vi "auto avance ralentir.vi"(9 "vitesse gauche":dbl, 10 "temps":dbl, 11 "temps de changement de direction":dbl) -> ()   [LabVIEW 2015]
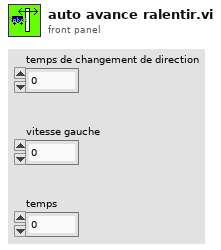
[diagram p1: front panel]
types:
  T1 = typedef "WPI_ServoDeviceRef.ctl" = cluster{"DeviceStatus":errorcluster, "PWM Channel":T2, "DeadBand":T3}
  T2 = typedef "FPGA_DIOPWMChannel.ctl" = enum8{"PWM 0", "PWM 1", "PWM 2", "PWM 3", "PWM 4", "PWM 5", "PWM 6", "PWM 7", "PWM 8", "PWM 9", "PWM MXP 0", "PWM MXP 1", "PWM MXP 2", "PWM MXP 3", "PWM MXP 4", "PWM MXP 5", "PWM MXP 6", "PWM MXP 7", "PWM MXP 8", "PWM MXP 9", "Invalid"}
  T3 = typedef "WPI_PWMDeadband.ctl" = cluster{"Name":string, "maxPositivePwm":i32, "minPositivePwm":i32, "centerPwm":i32, "maxNegativePwm":i32, "minNegativePwm":i32, "angularRange":u16}
  T4 = typedef "WPI_EncoderDevRef.ctl" = cluster{"DevStatus":errorcluster, "EncoderIndex":T5, "CounterIndex":T6, "DistancePerCount":dbl, "Decoding Type":T7}
  T5 = typedef "FPGA_EncoderIdx.ctl" = enum8{"Enc 0", "Enc 1", "Enc 2", "Enc 3", "Enc 4", "Enc 5", "Enc 6", "Enc 7", "Invalid"}
  T6 = typedef "FPGA_CounterCtrSystemIndex.ctl" = enum8{"Ctr 0", "Ctr 1", "Ctr 2", "Ctr 3", "Ctr 4", "Ctr 5", "Ctr 6", "Ctr 7", "Invalid"}
  T7 = typedef "WPI_EncoderType.ctl" = enum16{"1x", "2x", "4x"}
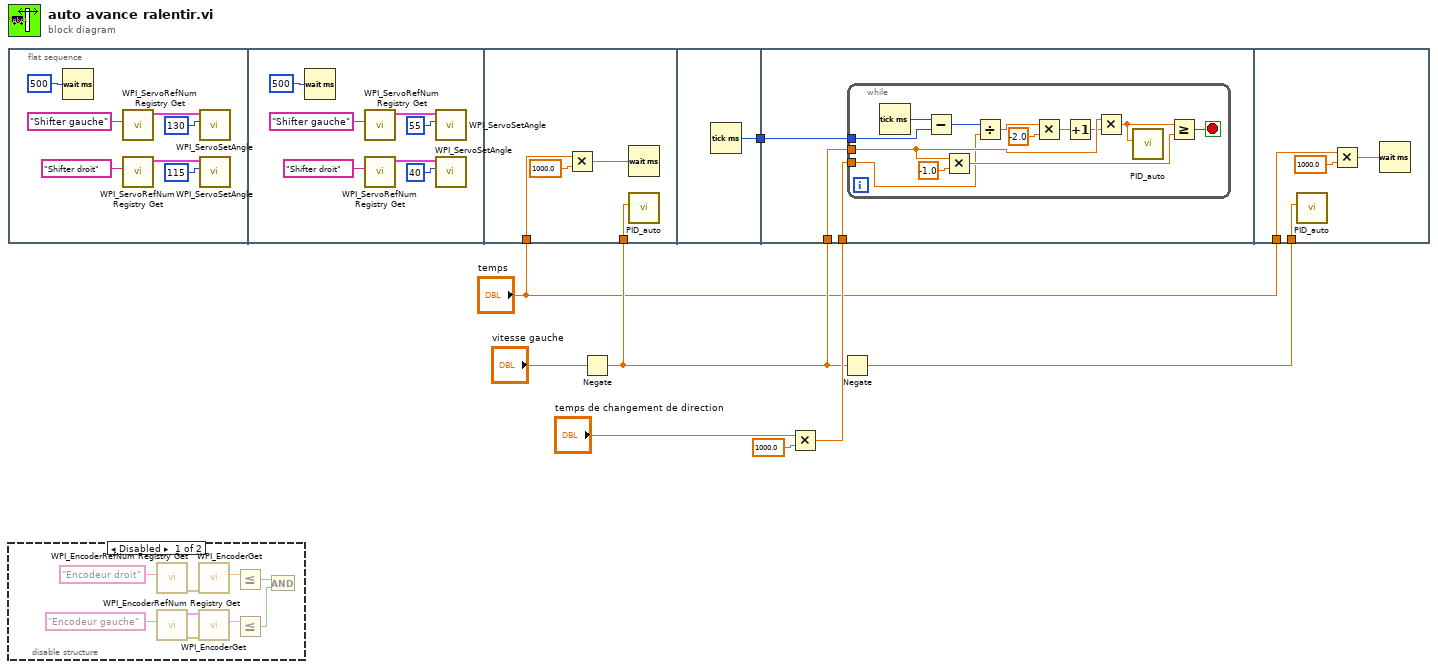
[diagram p0: block diagram]
diagram:
  n1 = flat-sequence {
    tunnel: w3 -> [w26]
    tunnel: "temps" -> [w24]
    tunnel: [w27] -> w8
    tunnel: w8 -> [w30]
    tunnel: w3 -> [w29]
    tunnel: w5 -> [w28]
    tunnel: w2 -> [w47]
    tunnel: "temps" -> [w44]
    frame #0 {
      n2 = Wait (ms)(milliseconds to wait=u32 500) -> ()  [unwired: 1 out]
      n3 = call <vilib>:"WPI_ServoRefNum Registry Get.vi"("refnum name"="Shifter gauche") -> ("ServoDeviceRef"=w14:T1)  [unwired: 9 in, 1 out]
      n4 = call <vilib>:"WPI_ServoRefNum Registry Get.vi"("refnum name"="Shifter droit") -> ("ServoDeviceRef"=w15:T1)  [unwired: 9 in, 1 out]
      n5 = call <vilib>:"WPI_ServoSetAngle.vi"("Angle"=130, "ServoDeviceRef"=w14) -> ()  [unwired: 8 in, 2 out]
      n6 = call <vilib>:"WPI_ServoSetAngle.vi"("Angle"=115, "ServoDeviceRef"=w15) -> ()  [unwired: 8 in, 2 out]
    }
    frame #1 {
      n7 = Wait (ms)(milliseconds to wait=u32 500) -> ()  [unwired: 1 out]
      n8 = call <vilib>:"WPI_ServoRefNum Registry Get.vi"("refnum name"="Shifter gauche") -> ("ServoDeviceRef"=w21:T1)  [unwired: 9 in, 1 out]
      n9 = call <vilib>:"WPI_ServoRefNum Registry Get.vi"("refnum name"="Shifter droit") -> ("ServoDeviceRef"=w22:T1)  [unwired: 9 in, 1 out]
      n10 = call <vilib>:"WPI_ServoSetAngle.vi"("Angle"=55, "ServoDeviceRef"=w21) -> ()  [unwired: 8 in, 2 out]
      n11 = call <vilib>:"WPI_ServoSetAngle.vi"("Angle"=40, "ServoDeviceRef"=w22) -> ()  [unwired: 8 in, 2 out]
    }
    frame #2 {
      n12 = Multiply(x=w24, y=1000.0) -> (x*y=w23:dbl)
      n13 = Wait (ms)(milliseconds to wait=w23) -> ()  [unwired: 1 out]
      n14 = call "PID_auto.vi"("vitesse voulu"=w26) -> ()  [unwired: 11 in]
    }
    frame #3 {
      n15 = Tick Count (ms)() -> (millisecond timer value=w27:u32)
    }
    frame #4 {
      n16 = while {
        tunnel: w30 -> [w34]
        tunnel: w29 -> [w42]
        tunnel: w28 -> [w40]
        stop <- w31 stop-if-true
        n17 = Tick Count (ms)() -> (millisecond timer value=w33:u32)
        n18 = Subtract(x=w33, y=w34) -> (x-y=w39:u32)
        n19 = Multiply(x=w42, y=-1.0) -> (x*y=w41:dbl)
        n20 = Divide(x=w39, y=w40) -> (x/y=w37:dbl)
        n21 = Multiply(x=w37, y=-2.0) -> (x*y=w36:dbl)
        n22 = Increment(x=w36) -> (x+1=w35:dbl)
        n23 = Multiply(x=w42, y=w35) -> (x*y=w32:dbl)
        n24 = call "PID_auto.vi"("vitesse voulu"=w32) -> ()  [unwired: 11 in]
        n25 = Greater Or Equal?(x=w32, y=w41) -> (x >= y?=w31:bool)
      }
    }
    frame #5 {
      n26 = call "PID_auto.vi"("vitesse voulu"=w47) -> ()  [unwired: 11 in]
      n27 = Multiply(x=w44, y=1000.0) -> (x*y=w46:dbl)
      n28 = Wait (ms)(milliseconds to wait=w46) -> ()  [unwired: 1 out]
    }
  }
  n29 = disable-structure shown="Disabled" {
    frame Disabled {
      n30 = call <vilib>:"WPI_EncoderRefNum Registry Get.vi"("refnum name"="Encodeur droit") -> ("error out"=w48:errorcluster)  [unwired: 9 in, 1 out]
      n31 = call <vilib>:"WPI_EncoderRefNum Registry Get.vi"("refnum name"="Encodeur gauche") -> ("error out"=w50:errorcluster, "EncoderDevRef"=w51:T4)  [unwired: 9 in]
      n32 = call <vilib>:"WPI_EncoderGet.vi"("error in (no error)"=w48) -> ("Distance"=w53:dbl)  [unwired: 5 in, 5 out]
      n33 = call <vilib>:"WPI_EncoderGet.vi"("error in (no error)"=w50, "EncoderDevRef"=w51) -> ("Distance"=w56:dbl)  [unwired: 4 in, 5 out]
      n34 = Less Or Equal?(x=w53) -> (x <= y?=w54:bool)  [unwired: 1 in]
      n35 = Less Or Equal?(x=w56) -> (x <= y?=w55:bool)  [unwired: 1 in]
      n36 = And(x=w54, y=w55) -> ()  [unwired: 1 out]
    }
    frame Enabled {
    }
  }
  n37 = Negate(x="vitesse gauche") -> (-x=w3:dbl)
  n38 = Multiply(x="temps de changement de direction", y=1000.0) -> (x*y=w5:dbl)
  n39 = Negate(x=w3) -> (-x=w2:dbl)
